vi "EditedPicoScope2000aOpen.vi"(4 "serial":i8[](array[numeric]), 7 "error in (no error)":errorcluster) -> (0 "Max Adc value":i16, 2 "handle":i16, 3 "error out":errorcluster, 5 "Device Info":T1)   [LabVIEW 2024]
doc: "This VI opens a PicoScope 3000a/b and returns a handle to the device."
uses:
  ps2000a.dll
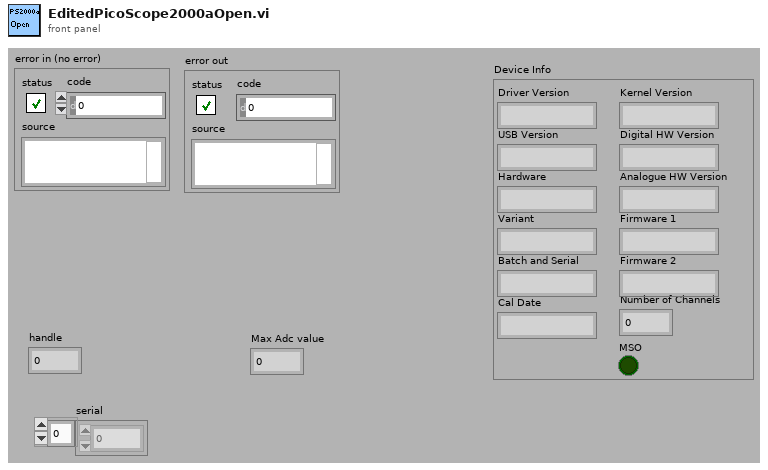
[diagram p1: front panel]
types:
  T1 = cluster{"Driver Version":string, "USB Version":string, "Hardware":string, "Variant":string, "Batch and Serial":string, "Cal Date":string, "Kernel Version":string, "Digital HW Version":string, "Analogue HW Version":string, "Firmware 1":string, "Firmware 2":string, "MSO":bool, "Number of Channels":i16}
  T2 = cluster{"Driver Version":string, "USB Version":string, "Hardware":string, "Variant":string, "Batch and Serial":string, "Cal Date":string, "Kernel Version":string, "Digital HW Version":string, "Analogue HW Version":string, "Firmware 1":string, "Firmware 2":string}
  T3 = cluster{"Driver Version":string, "USB Version":string, "Hardware":string, "Variant":string, "Batch and Serial":string, "Cal Date":string, "Kernel Version":string, "Digital HW Version":string, "Analogue HW Version":string, "Firmware 1":string, "Firmware 2":string, bool, i16}
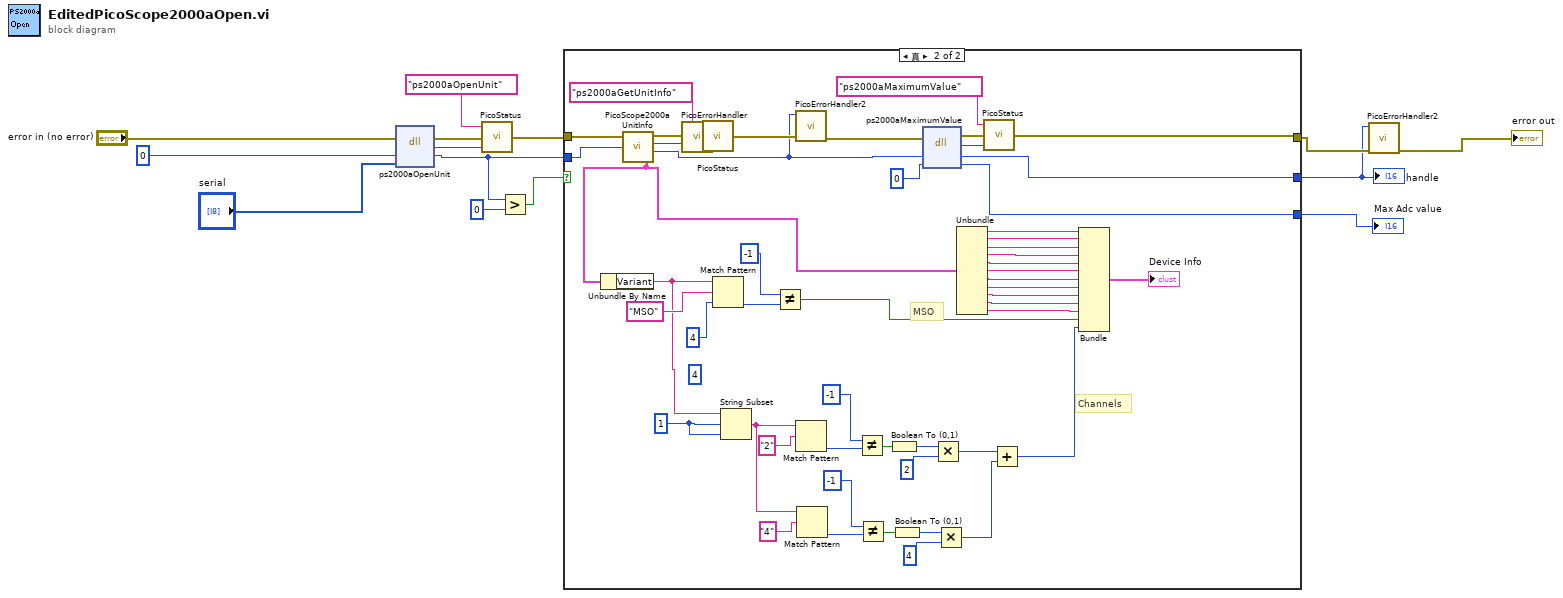
[diagram p0: block diagram]
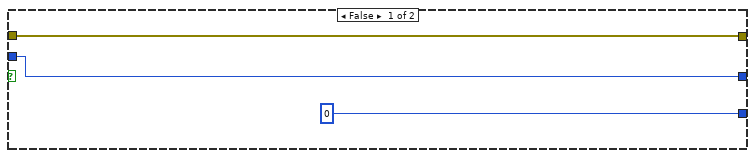
[diagram p2: hidden frame]
diagram:
  n1 = dll-call lib="ps2000a.dll" fn="ps2000aOpenUnit" ("ps3000.dll:_ps3000_open_unit@0")(error in="error in (no error)", "handle"=i16 0, "serial"="serial") -> (error out=w6:errorcluster, "PICO_STATUS"=w3:u32, "handle"=w2:i16)  [unwired: 3 in, 1 out]
  n2 = call "PicoStatus.vi"("PICO STATUS"=w3, "error in"=w6, "source"="ps2000aOpenUnit") -> ("error out"=w11:errorcluster)
  n3 = Greater?(x=w2, y=i16 0) -> (0:w13:bool)
  n4 = case shown="真" w13 {
    tunnel: w2 -> [w16 w66]
    tunnel: w11 -> [w17 w67]
    tunnel: [w17 w21] -> w9
    tunnel: [w16 w62] -> w7
    tunnel: [i16 0 ("value") w63] -> w10
    frame False {
    }
    frame True {
      w40 = 1 ("offset (0)")
      (unwired) 4 ("offset (0)")
      # "MSO"
      # "Channels"
      n5 = call "PicoScope2000aUnitInfo.vi"("error in (no error)"=w67, "handle in"=w66) -> ("error out"=w65:errorcluster, "PICO_STATUS"=w64:u32, "handle out"=w18:i16, "Unit Info"=w52:T2)  [unwired: 1 in]
      n6 = Unbundle By Name(w52) -> ("Variant"=w24:string)
      n7 = call "PicoStatus.vi"("PICO STATUS"=w64, "error in"=w65, "source"="ps2000aGetUnitInfo") -> ("error out"=w20:errorcluster)
      n8 = Match Pattern(string=w24, regular expression="MSO", offset (0)=4) -> (offset past match=w56:i32)  [unwired: 3 out]
      n9 = String Subset(string=w24, offset (0)=w40, length (rest)=w40) -> (substring=w33:string)
      n10 = Not Equal?(x=-1, y=w56) -> (x != y?=w53:bool)
      n11 = call "PicoErrorHandler2.vi"("error in (no error)"=w20, "handle In"=w18) -> ("error out"=w19:errorcluster)  [unwired: 9 in]
      n12 = Match Pattern(string=w33, regular expression="2") -> (offset past match=w38:i32)  [unwired: 1 in, 3 out]
      n13 = Match Pattern(string=w33, regular expression="4") -> (offset past match=w35:i32)  [unwired: 1 in, 3 out]
      n14 = Not Equal?(x=-1, y=w38) -> (x != y?=w30:bool)
      n15 = Not Equal?(x=-1, y=w35) -> (x != y?=w26:bool)
      n16 = Boolean To (0,1)(Boolean=w30) -> (0, 1=w29:i16)
      n17 = Boolean To (0,1)(Boolean=w26) -> (0, 1=w27:i16)
      n18 = dll-call lib="ps2000a.dll" fn="ps2000aMaximumValue"(error in=w19, "handle"=w18, "value"=i16 0) -> (error out=w60:errorcluster, "PICO_STATUS"=w59:u32, "handle"=w62:i16, "value"=w63:i16)  [unwired: 2 in, 1 out]
      n19 = Multiply(x=w29, y=i16 2) -> (x*y=w32:i16)
      n20 = Multiply(x=w27, y=i16 4) -> (x*y=w25:i16)
      n21 = Unbundle(w52) -> ("Driver Version"=w41:string, "USB Version"=w42:string, "Hardware"=w43:string, "Variant"=w44:string, "Batch and Serial"=w45:string, "Cal Date"=w46:string, "Kernel Version"=w47:string, "Digital HW Version"=w48:string, "Analogue HW Version"=w49:string, "Firmware 1"=w50:string, "Firmware 2"=w51:string)
      n22 = call "PicoStatus.vi"("PICO STATUS"=w59, "error in"=w60, "source"="ps2000aMaximumValue") -> ("error out"=w21:errorcluster)
      n23 = Add(x=w32, y=w25) -> (x+y=w23:i16)
      n24 = Bundle("Driver Version"=w41, "USB Version"=w42, "Hardware"=w43, "Variant"=w44, "Batch and Serial"=w45, "Cal Date"=w46, "Kernel Version"=w47, "Digital HW Version"=w48, "Analogue HW Version"=w49, "Firmware 1"=w50, "Firmware 2"=w51, w53, w23) -> (→"Device Info":T3)  [unwired: 1 in]
    }
  }
  "handle" <- w7
  "Max Adc value" <- w10
  n25 = call "PicoErrorHandler.vi"() -> ()  [unwired: 1 in, 1 out]
  n26 = call "PicoErrorHandler2.vi"("error in (no error)"=w9, "handle In"=w7) -> ("error out"=→"error out":errorcluster)  [unwired: 9 in]
